vi "SMO.jsonRPC.TestLauncher.vi"() -> ()   [LabVIEW 2013, in "SMO.jsonRPC.lvclass"]
doc: "JKI State Machine Objects (SMO) 1.0.0.5\nJKI - JKI\nCopyright (c) 2016, JKI"
uses:
  SMO.jsonRPC.lvclass
  <vilib>/JKI/JKI SMO/SMO/Typedefs/SMOState --Enum.ctl
  <vilib>/JKI/JKI SMO/SMO/SMO.lvclass
panel:
  out "id":i32
  in  "Send Async":bool
  out "Sync Response":string
  out "Async Response":variant
  in  "Send Sync":bool
  in  "Request parameters":string
  out "last error":errorcluster
  in  "Stop":bool
  # "JSON-RPC based messages Test Launcher"
  # "For instructions on how to use the JKI State Machine Objects, examples and video tutorials, visit:\nhttp://jki.net/state-machine-objects/\n\nJKI State Machine Objects™\nhttp://jki.net/state-machine-objects/\nCopyright (C) 2005-2015, JKI <info@jki.net>\nALL RIGHTS RESERVED"
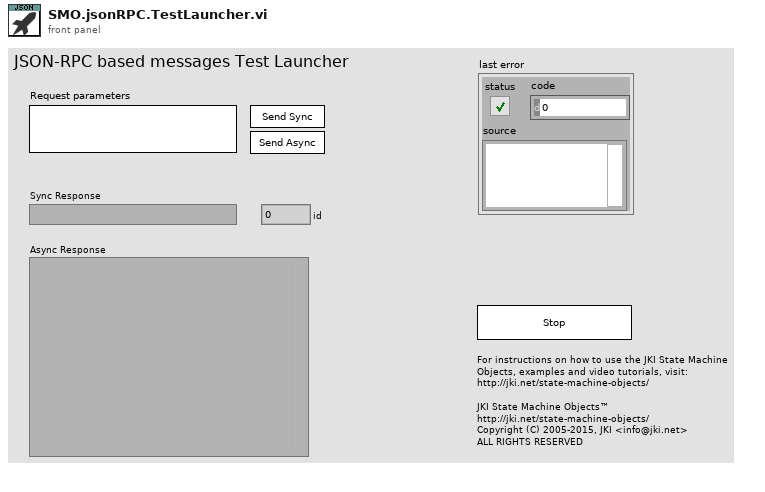
[diagram p1: front panel]
types:
  T1 = typedef "SMO.jsonRPC.lvclass/PublicEvents--Cluster.ctl" = cluster{"Reply":refnum<user-event>}
  T2 = typedef "SMO.lvclass/Public Events.ctl" = cluster{"Error":refnum<user-event>, "State":refnum<user-event>}
  T3 = typedef "SMO.lvclass/SMOState --Enum.ctl" = enum16{"unknown", "Created", "Started", "Stopped"}
  T4 = cluster{"Request parameters":string, "number: 0 to 1":dbl, bool}
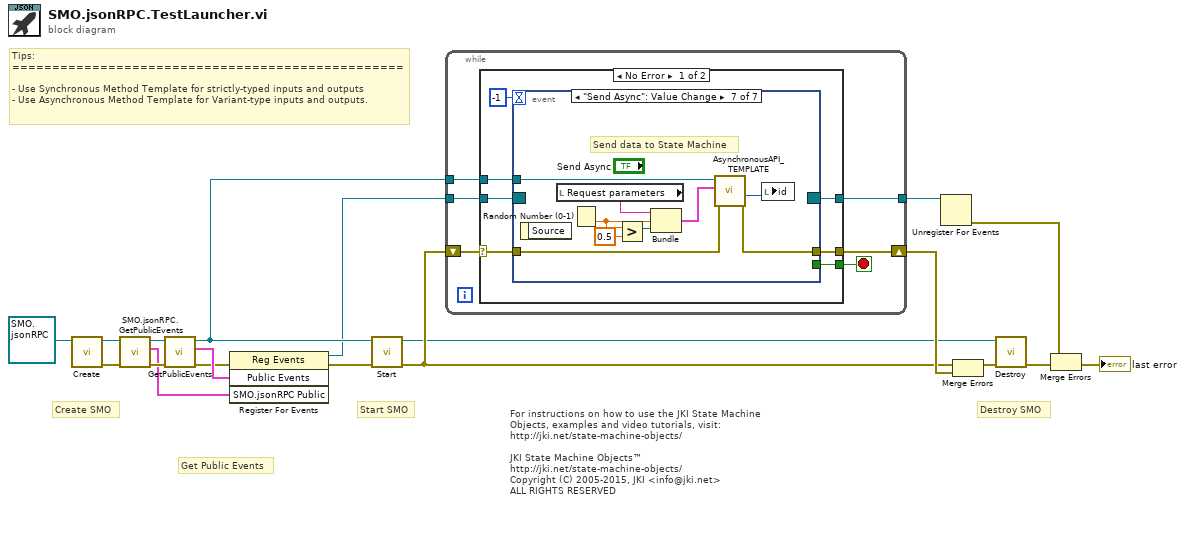
[diagram p0: block diagram]
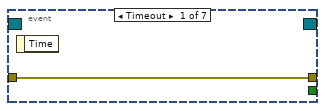
[diagram p2: hidden frame]
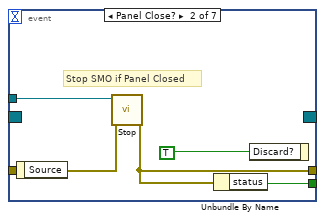
[diagram p3: hidden frame]
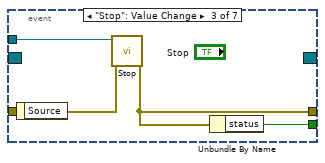
[diagram p4: hidden frame]
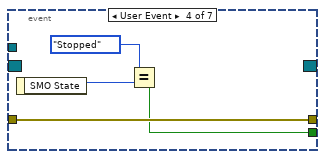
[diagram p5: hidden frame]
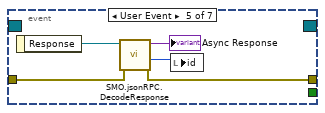
[diagram p6: hidden frame]
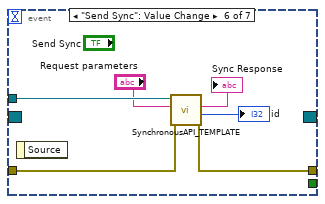
[diagram p7: hidden frame]
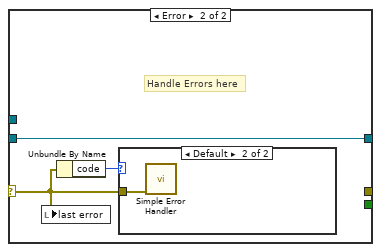
[diagram p8: hidden frame]
diagram:
  # "Tips: \n=================================================\n\n- Use Synchronous Method Template for strictly-typed inputs and outputs\n- Use Asynchronous Method Template for Variant-type inputs and outputs."
  # "For instructions on how to use the JKI State Machine Objects, examples and video tutorials, visit:\nhttp://jki.net/state-machine-objects/\n\nJKI State Machine Objects™\nhttp://jki.net/state-machine-objects/\nCopyright (C) 2005-2015, JKI <info@jki.net>\nALL RIGHTS RESERVED"
  # "Get Public Events"
  # "Start SMO"
  # "Destroy SMO"
  # "Create SMO"
  n1 = call <vilib>:"Create.vi"("SMO"=refnum<class "SMO.jsonRPC.lvclass"> refnum ("SMO.Template.lvclass")) -> ("error out"=w5:errorcluster, "SMO out"=w3:refnum<class "SMO.jsonRPC.lvclass">)  [unwired: 8 in, 1 out]
  n2 = call "SMO.jsonRPC.GetPublicEvents.vi"("error in (no error)"=w5, "SMO.jsonRPC"=w3) -> ("error out"=w4:errorcluster, "SMO.jsonRPC Public"=w1:T1, "SMO.jsonRPC out"=w2:refnum<class "SMO.jsonRPC.lvclass">)  [unwired: 7 in]
  n3 = call <vilib>:"GetPublicEvents.vi"("error in (no error)"=w4, "SMO"=w2) -> ("error out"=w7:errorcluster, "Public Events"=w8:T2, "SMO out"=w10:refnum<class "SMO.jsonRPC.lvclass">)  [unwired: 7 in]
  n4 = register-events(error in=w7, w8, w1) -> (reference out=w6:refnum<event-registration>, error out=w9:errorcluster)  [unwired: 1 in]
  n5 = call <vilib>:"Start.vi"("error in (no error)"=w9, "SMO"=w10) -> ("error out"=w13:errorcluster, "SMO out"=w11:refnum<class "SMO.jsonRPC.lvclass">)  [unwired: 8 in]
  n6 = while {
    shift-right: [w24] -> w18
    shift-left: w13 -> [w20]
    tunnel: w6 -> [w23]
    tunnel: [w22] -> w19
    tunnel: w10 -> [w21]
    stop <- w25 stop-if-true
    n7 = case shown="No Error" w20 {
      selector: w20 -> [w26 w67]
      tunnel: [w32 _] -> w25
      tunnel: [w31 _] -> w24
      tunnel: w23 -> [w30 w69]
      tunnel: [w29 w69] -> w22
      tunnel: w21 -> [w28 _]
      frame No Error {
        n8 = event shown="[6] \"Send Async\": Value Change" {
          selector: w30 -> [_ _ _ _ _ _ _]
          dyn-events: [_ _ _ _ _ _ _] -> w29
          timeout: -1 -> [_ _ _ _ _ _ _]
          tunnel: [_ w34 w39 w43 _ _ _] -> w32
          tunnel: w28 -> [_ w38 w42 _ _ w57 w66]
          tunnel: [w33 w35 w40 w46 w49 w54 w64] -> w31
          tunnel: w26 -> [w33 w37 w41 w46 w50 w55 w65]
          event Timeout {
            n9 = event-data() -> ()  [unwired: 1 in, 1 out]
          }
          event Panel Close? {
            # "Stop SMO if Panel Closed"
            n10 = event-data() -> ()  [unwired: 1 in, 1 out]
            n11 = call <vilib>:"Stop.vi"("error in (no error)"=w37, "SMO"=w38) -> ("error out"=w35:errorcluster)  [unwired: 8 in, 1 out]
            n12 = Unbundle By Name(w35) -> ("status"=w34:bool)
            n13 = event-data("Discard?"=TRUE ("OK")) -> ()  [unwired: 1 in, 1 out]
          }
          event "Stop": Value Change {
            n14 = event-data() -> ()  [unwired: 1 in, 1 out]
            n15 = call <vilib>:"Stop.vi"("error in (no error)"=w41, "SMO"=w42) -> ("error out"=w40:errorcluster)  [unwired: 8 in, 1 out]
            n16 = Unbundle By Name(w40) -> ("status"=w39:bool)
          }
          event User Event {
            n17 = event-data() -> ("SMO State"=w45:T3)  [unwired: 1 in]
            n18 = Equal?(x=SMOState_--Enum."Stopped", y=w45) -> (x = y?=w43:bool)
          }
          event User Event {
            n19 = event-data() -> ("Response"=w51:refnum<class "Response.lvclass">)  [unwired: 1 in]
            n20 = call "SMO.jsonRPC.DecodeResponse.vi"("error in (no error)"=w50, "jsonRPC response"=w51) -> ("error out"=w49:errorcluster, "id"=w47:i32, "result"=→"Async Response":variant)  [unwired: 7 in]
            n21 = local write "id"(w47) -> ()
          }
          event "Send Sync": Value Change {
            n22 = event-data() -> ()  [unwired: 1 in, 1 out]
            n23 = call "SynchronousAPI_TEMPLATE.vi"("error in (no error)"=w55, "myData"="Request parameters", "SMO.jsonRPC"=w57) -> ("error out"=w54:errorcluster, "id"=→"id":i32, "reply"=→"Sync Response":string)  [unwired: 5 in, 1 out]
          }
          event "Send Async": Value Change {
            # "Send data to State Machine"
            n24 = event-data() -> ()  [unwired: 1 in, 1 out]
            n25 = local read "Request parameters"() -> (w58:string)
            n26 = Random Number (0-1)() -> (number: 0 to 1=w60:dbl)
            n27 = Greater?(x=w60, y=0.5) -> (0:w59:bool)
            n28 = Bundle("Request parameters"=w58, "number: 0 to 1"=w60, w59) -> (w61:T4)  [unwired: 1 in]
            n29 = call "AsynchronousAPI_TEMPLATE.vi"("error in (no error)"=w65, "Parameters"=w61, "SMO.jsonRPC"=w66) -> ("error out"=w64:errorcluster, "id"=w63:i32)  [unwired: 6 in, 1 out]
            n30 = local write "id"(w63) -> ()
          }
        }
      }
      frame Error {
        # "Handle Errors here"
        n31 = local write "last error"(w67) -> ()
        n32 = Unbundle By Name(w67) -> ("code"=w68:i32)
        n33 = case shown="Default" w68 {
          tunnel: w67 -> [_ w70]
          frame 0 {
          }
          frame Default {
            n34 = call <vilib>:"Simple Error Handler.vi"("error in (no error)"=w70) -> ()  [unwired: 4 in, 5 out]
          }
        }
      }
    }
  }
  n35 = Unregister For Events(event registration refnum=w19) -> (error out=w17:errorcluster)  [unwired: 1 in]
  n36 = Merge Errors(w13, w18) -> (w12:errorcluster)
  n37 = call <vilib>:"Destroy.vi"("error in (no error)"=w12, "SMO"=w11) -> ("error out"=w15:errorcluster)  [unwired: 9 in]
  n38 = Merge Errors(w17, w15) -> (→"last error":errorcluster)
